vi "Init Edge Detection.vi"(8 "error in (no error)":errorcluster, 9 "Last output":dbl, 10 "First output":dbl, 11 "RP Transceiver in":refnum<class "RP Transceiver.lvclass">) -> (0 "error out":errorcluster, 3 "RP Transceiver out":refnum<class "RP Transceiver.lvclass">)   [LabVIEW 2016, in "RP Transceiver.lvclass"]
uses:
  RP Transceiver.lvclass
  RP Transceiver.lvclass/RP Transceiver.ctl
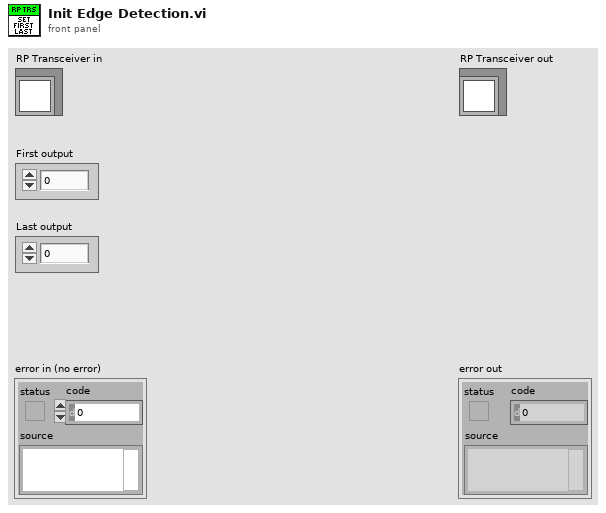
[diagram p1: front panel]
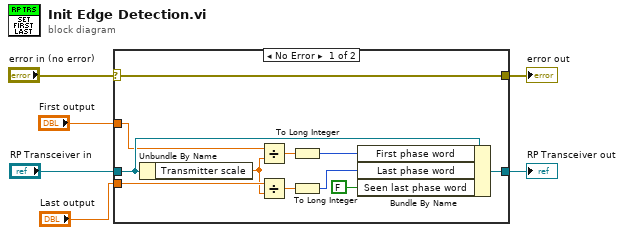
[diagram p0: block diagram]
diagram:
  n1 = case shown="No Error" "error in (no error)" {
    selector: "error in (no error)" -> [w17 w19]
    tunnel: [w17 w19] -> w5
    tunnel: [w12 w18] -> w3
    tunnel: "RP Transceiver in" -> [w16 w18]
    tunnel: "First output" -> [w15 _]
    tunnel: "Last output" -> [w14 _]
    frame No Error {
      n2 = Unbundle By Name(w16) -> ("Transmitter scale"=w13:dbl)
      n3 = Divide(x=w15, y=w13) -> (x/y=w11:dbl)
      n4 = Divide(x=w14, y=w13) -> (x/y=w10:dbl)
      n5 = To Long Integer(number=w11) -> (32bit integer=w9:i32)
      n6 = To Long Integer(number=w10) -> (32bit integer=w8:i32)
      n7 = Bundle By Name(cluster=w16, "First phase word"=w9, "Last phase word"=w8, "Seen last phase word"=FALSE) -> (w12:refnum<class "RP Transceiver.lvclass">)
    }
    frame Error {
    }
  }
  "error out" <- w5
  "RP Transceiver out" <- w3
